vi "Vision Center.vi"(0 "Intake":dbl=1.0, 1 "X axis value":dbl=0.05 format="%#_13g", 2 "X axis value 2":dbl=-0.05) -> ()   [LabVIEW 2015]
uses:
  Robot Global Data.vi
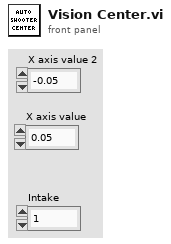
[diagram p1: front panel]
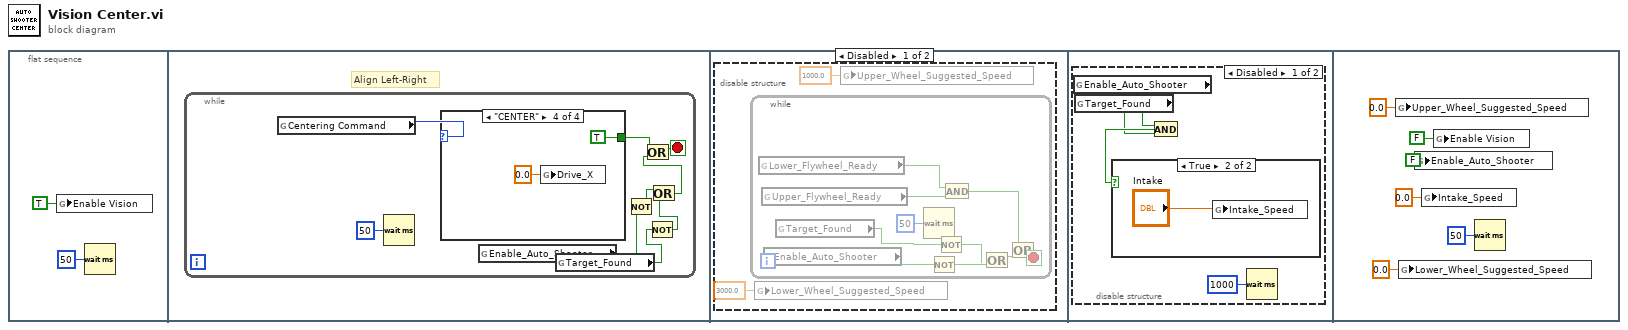
[diagram p0: block diagram]
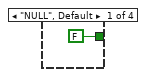
[diagram p2: hidden frame]
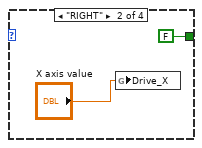
[diagram p3: hidden frame]
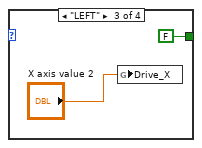
[diagram p4: hidden frame]
diagram:
  n1 = flat-sequence {
    frame #0 {
      n2 = global write "Robot Global Data.vi" "Enable Vision"(TRUE ("Enable Vision")) -> ()
      n3 = Wait (ms)(milliseconds to wait=u32 50) -> ()  [unwired: 1 out]
    }
    frame #1 {
      # "Align Left-Right"
      n4 = while {
        stop <- w8 stop-if-true
        n5 = global read "Robot Global Data.vi" "Centering Command"() -> (w10:enum16{"NULL", "RIGHT", "LEFT", "CENTER"})
        n6 = Wait (ms)(milliseconds to wait=u32 50) -> ()  [unwired: 1 out]
        n7 = case shown="\"CENTER\"" w10 {
          tunnel: [FALSE FALSE FALSE TRUE] -> w11
          frame "NULL", Default {
          }
          frame "RIGHT" {
            n8 = global write "Robot Global Data.vi" "Drive_X"("X axis value") -> ()
          }
          frame "LEFT" {
            n9 = global write "Robot Global Data.vi" "Drive_X"("X axis value 2") -> ()
          }
          frame "CENTER" {
            n10 = global write "Robot Global Data.vi" "Drive_X"(0.0 ("Drive_X")) -> ()
          }
        }
        n11 = global read "Robot Global Data.vi" "Enable_Auto_Shooter"() -> (w7:bool)
        n12 = global read "Robot Global Data.vi" "Target_Found"() -> (w5:bool)
        n13 = Not(x=w7) -> (.not. x?=w6:bool)
        n14 = Not(x=w5) -> (.not. x?=w4:bool)
        n15 = Or(x=w6, y=w4) -> (x .or. y?=w3:bool)
        n16 = Or(x=w11, y=w3) -> (x .or. y?=w8:bool)
      }
    }
    frame #2 {
      n17 = disable-structure shown="Disabled" {
        frame Disabled {
          n18 = while {
            stop <- w26 stop-if-true
            n19 = global read "Robot Global Data.vi" "Lower_Flywheel_Ready"() -> (w29:bool)
            n20 = global read "Robot Global Data.vi" "Upper_Flywheel_Ready"() -> (w30:bool)
            n21 = global read "Robot Global Data.vi" "Enable_Auto_Shooter"() -> (w25:bool)
            n22 = global read "Robot Global Data.vi" "Target_Found"() -> (w22:bool)
            n23 = Wait (ms)(milliseconds to wait=u32 50) -> ()  [unwired: 1 out]
            n24 = Not(x=w25) -> (.not. x?=w24:bool)
            n25 = Not(x=w22) -> (.not. x?=w21:bool)
            n26 = And(x=w29, y=w30) -> (x .and. y?=w28:bool)
            n27 = Or(x=w24, y=w21) -> (x .or. y?=w23:bool)
            n28 = Or(x=w28, y=w23) -> (x .or. y?=w26:bool)
          }
          n29 = global write "Robot Global Data.vi" "Lower_Wheel_Suggested_Speed"(3000.0 ("Lower_Wheel_Suggested_Speed")) -> ()
          n30 = global write "Robot Global Data.vi" "Upper_Wheel_Suggested_Speed"(1000.0 ("Upper_Wheel_Suggested_Speed")) -> ()
        }
        frame Enabled {
        }
      }
    }
    frame #3 {
      n31 = disable-structure shown="Disabled" {
        frame Disabled {
          n32 = global read "Robot Global Data.vi" "Enable_Auto_Shooter"() -> (w33:bool)
          n33 = global read "Robot Global Data.vi" "Target_Found"() -> (w31:bool)
          n34 = And(x=w33, y=w31) -> (x .and. y?=w32:bool)
          n35 = case shown="True" w32 {
            frame False {
            }
            frame True {
              n36 = global write "Robot Global Data.vi" "Intake_Speed"("Intake") -> ()
            }
          }
          n37 = Wait (ms)(milliseconds to wait=u32 1000) -> ()  [unwired: 1 out]
        }
        frame Enabled {
        }
      }
    }
    frame #4 {
      n38 = global write "Robot Global Data.vi" "Upper_Wheel_Suggested_Speed"(0.0 ("Upper_Wheel_Suggested_Speed")) -> ()
      n39 = global write "Robot Global Data.vi" "Lower_Wheel_Suggested_Speed"(0.0 ("Lower_Wheel_Suggested_Speed")) -> ()
      n40 = global write "Robot Global Data.vi" "Enable_Auto_Shooter"(FALSE ("Enable_Shooter")) -> ()
      n41 = global write "Robot Global Data.vi" "Intake_Speed"(0.0 ("Intake_Speed")) -> ()
      n42 = global write "Robot Global Data.vi" "Enable Vision"(FALSE ("Enable Vision")) -> ()
      n43 = Wait (ms)(milliseconds to wait=u32 50) -> ()  [unwired: 1 out]
    }
  }
